vi "Score Particles.vi"(8 "Area Size Limit":i32=444, 9 "Particle Count Limit":i32=10, 11 "Image Refnum in":T1) -> (2 "Scored Particle Info":T2(array[cluster]), 3 "Image Refnum out":T1)   [LabVIEW 2013]
doc: "Score the largest particles in the image to determine how well they match the target attributes. Specifically, calculate how rectangular a particle is, inspect its aspect ratio, and determine if it is hollow (having pixels on around the edges, but off in the large center)."
uses:
  <vilib>/vision/NI_Vision_Development_Module.lvlib
  <vilib>/vision/Image Controls.llb/IMAQ Image.ctl
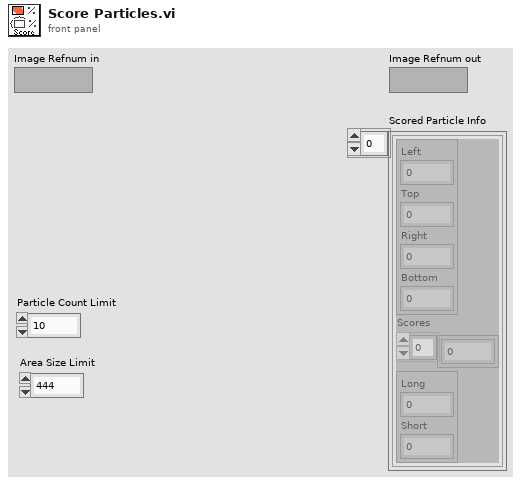
[diagram p1: front panel]
types:
  T1 = typedef "IMAQ Image.ctl" = refnum<image>
  T2 = cluster{cluster{"Left":dbl, "Top":dbl, "Right":dbl, "Bottom":dbl}, "Scores":dbl[], cluster{"Long":dbl, "Short":dbl}}[]
  T3 = typedef "Particle Parameters" = i32
  T4 = typedef "Image Type" = u32
  T5 = cluster{"Left":dbl, "Top":dbl, "Right":dbl, "Bottom":dbl}
  T6 = cluster{cluster{"Left":dbl, "Top":dbl, "Right":dbl, "Bottom":dbl}, dbl[], cluster{"Numeric":dbl, "Numeric":dbl}}
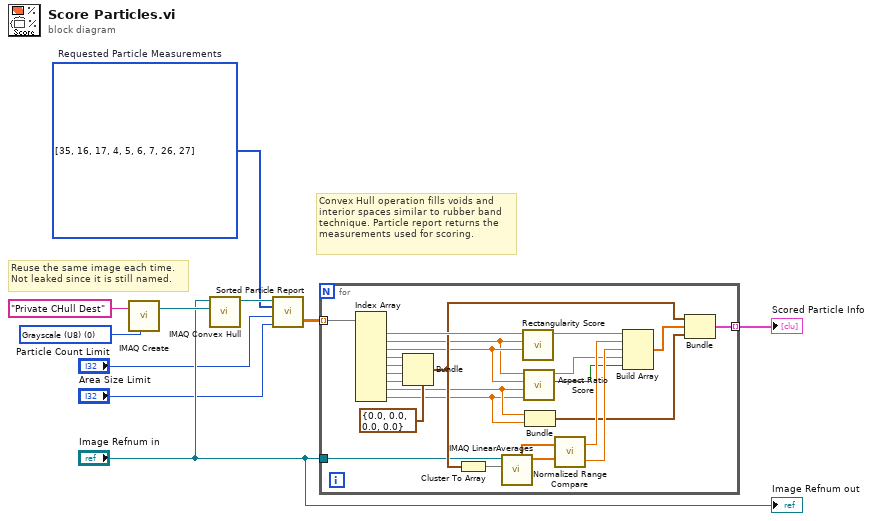
[diagram p0: block diagram]
diagram:
  w1 = T3[] [35, 16, 17, 4, 5, 6, 7, 26, 27] items=["Center of Mass X", "Center of Mass Y", "First Pixel X", "First Pixel Y", "Bounding Rect Left", "Bounding Rect Top", "Bounding Rect Right", "Bounding Rect Bottom", "Max Feret Diameter Start X", "Max Feret Diameter Start Y", "Max Feret Diameter End X", "Max Feret Diameter End Y", "Max Horiz. Segment Length Left", "Max Horiz. Segment Length Right", "Max Horiz. Segment Length Row", "-", "Bounding Rect Width", "Bounding Rect Height", "Bounding Rect Diagonal", "Perimeter", "Convex Hull Perimeter", "Holes' Perimeter", "Max Feret Diameter", "Equivalent Ellipse Major Axis", "Equivalent Ellipse Minor Axis", "Equivalent Ellipse Minor Axis (Feret)", "Equivalent Rect Long Side", "Equivalent Rect Short Side", "Equivalent Rect Diagonal", "Equivalent Rect Short Side (Feret)", "Average Horiz. Segment Length", "Average Vert. Segment Length", "Hydraulic Radius", "Waddel Disk Diameter", "-", "Area", "Holes' Area", "Particle & Holes' Area", "Convex Hull Area", "Image Area", "-", "Number of Holes", "Number of Horiz. Segments", "Number of Vert. Segments", "-", "Orientation", "Max Feret Diameter Orientation", "-", "% Area/Image Area", "% Area/(Particle & Holes' Area)", "Ratio of Equivalent Ellipse Axes", "Ratio of Equivalent Rect Sides", "-", "Elongation Factor", "Compactness Factor", "Heywood Circularity Factor", "Type Factor", "-", "Sum X", "Sum Y", "Sum XX", "Sum XY", "Sum YY", "Sum XXX", "Sum XXY", "Sum XYY", "Sum YYY", "-", "Moment of Inertia XX", "Moment of Inertia XY", "Moment of Inertia YY", "Moment of Inertia XXX", "Moment of Inertia XXY", "Moment of Inertia XYY", "Moment of Inertia YYY", "Norm. Moment of Inertia XX", "Norm. Moment of Inertia XY", "Norm. Moment of Inertia YY", "Norm. Moment of Inertia XXX", "Norm. Moment of Inertia XXY", "Norm. Moment of Inertia XYY", "Norm. Moment of Inertia YYY", "Hu Moment 1", "Hu Moment 2", "Hu Moment 3", "Hu Moment 4", "Hu Moment 5", "Hu Moment 6", "Hu Moment 7"]  # Requested Particle Measurements
  w7 = T4 0 items=["Grayscale (U8)", "Grayscale (I16)", "Grayscale (SGL)", "Complex (CSG)", "RGB (U32)", "HSL (U32)", "RGB (U64)", "Grayscale (U16)"] ("Image Type")
  # "Reuse the same image each time.\nNot leaked since it is still named."
  # "Convex Hull operation fills voids and\ninterior spaces similar to rubber band\ntechnique. Particle report returns the\nmeasurements used for scoring."
  n1 = call "IMAQ Create"("Image Name"="Private CHull Dest", "Image Type"=w7) -> ("New Image"=w6:T1)  [unwired: 2 in, 2 out]
  n2 = call "IMAQ Convex Hull"("Image Dst"=w6, "Image Src"="Image Refnum in") -> ("Image Dst Out"=w4:T1)  [unwired: 2 in, 7 out]
  n3 = call "Sorted Particle Report.vi"("Area Size Limit"="Area Size Limit", "Particle Count Limit"="Particle Count Limit", "Pixel Measurements"=w1, "Image in"=w4) -> ("Sorted Data"=w9:dbl[][])  [unwired: 1 out]
  n4 = for {
    tunnel: [w32] -> w10 mode=indexing
    tunnel: "Image Refnum in" -> [w26]
    tunnel: w9 -> [w25] mode=indexing
    n5 = Index Array(array=w25) -> (element #1=w33:dbl, element #2=w19:dbl, element #3=w20:dbl, element #4=w21:dbl, element #5=w22:dbl, element #6=w23:dbl, element #7=w24:dbl, element #8=w13:dbl, element #9=w12:dbl)  [unwired: 9 in]
    n6 = Bundle(cluster=T5 {"Left"=0.0, "Top"=0.0, "Right"=0.0, "Bottom"=0.0}, "Left"=w21, "Top"=w22, "Right"=w23, "Bottom"=w24) -> (w31:T5)
    n7 = Cluster To Array(cluster=w31) -> (array=w27:dbl[])
    n8 = call "IMAQ LinearAverages"("Optional Rectangle"=w27, "Image Src"=w26) -> ("Y Axis Averages"=w29:sgl[], "X Axis Averages"=w28:sgl[])  [unwired: 2 in, 6 out]
    n9 = call "Rectangularity Score.vi"("Height"=w20, "Width"=w19, "Area"=w33) -> ("Score"=w30:dbl)  [unwired: 8 in]
    n10 = call "Aspect Ratio Score.vi"("Equivalent Rect Short"=w12, "Equivalent Rect Long"=w13, "Height"=w20, "Width"=w19) -> ("Horizontal"=w15:bool, "Score"=w16:dbl)  [unwired: 6 in]
    n11 = Bundle("Numeric"=w13, "Numeric"=w12) -> (w11:cluster{"Numeric":dbl, "Numeric":dbl})  [unwired: 1 in]
    n12 = call "Normalized Range Compare.vi"("Y Averages"=w29, "X Averages"=w28) -> ("Y Score"=w17:dbl, "X Score"=w18:dbl)
    n13 = Build Array(w30, w18, w17, w16, w15) -> (w14:dbl[])
    n14 = Bundle(w31, w14, w11) -> (w32:T6)  [unwired: 1 in]
  }
  "Scored Particle Info" <- w10
  "Image Refnum out" <- "Image Refnum in"
